vi "infofile beta.vi"(6 "Info in":string[](array[string]), 7 "reference":refnum<vi>) -> (2 "String":string)   [LabVIEW 2020]
uses:
  <vilib>/Utility/Data Type/NI_Data Type.lvlib
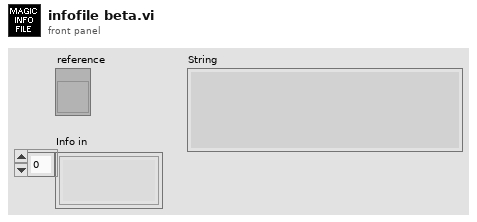
[diagram p1: front panel]
types:
  T1 = typedef "NI_Data Type.lvlib/Data Type.ctl" = enum8{"Invalid Type", "Void", "I8", "I16", "I32", "I64", "U8", "U16", "U32", "U64", "Single Float", "Double Float", "Extended Float", "Single Complex", "Double Complex", "Extended Complex", "Enum U8", "Enum U16", "Enum U32", "Enum U64", "Single Float With Unit", "Double Float With Unit", "Extended Float With Unit", "Single Complex with Unit", "Double Complex with Unit", "Extended Complex with Unit", "Boolean", "String", "Path", "Picture", "Tag", "Array", "Cluster", "Variant", "LV Variant", "Waveform", "Timestamp", "Digital Waveform", "Digital Data", "ExpressData", "Refnum", "External Data", "VI", "Poly VI", "LabVIEW Class Instance", "Fixed Point", "Set Collection", "Map Collection"}
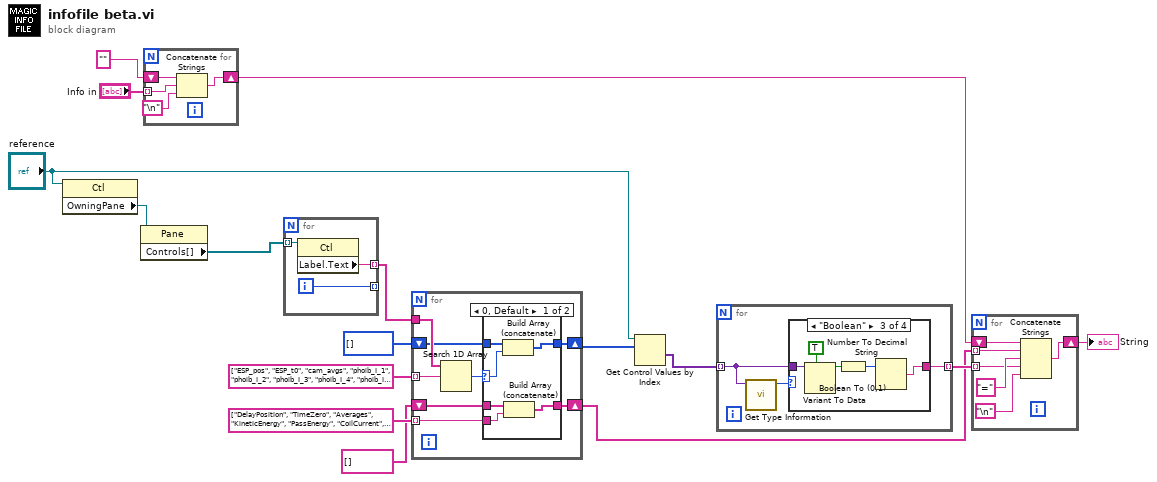
[diagram p0: block diagram]
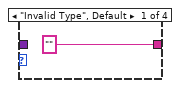
[diagram p2: hidden frame]
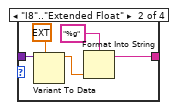
[diagram p3: hidden frame]
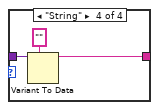
[diagram p4: hidden frame]
diagram:
  n1 = property class="Ctl"(reference="reference") -> ("OwningPane"=w2:refnum<vi>)  [unwired: 1 in, 2 out]
  n2 = property class="Pane"(reference=w2) -> ("Controls[]"=w1:refnum<vi>[])  [unwired: 1 in, 2 out]
  n3 = for {
    tunnel: "Info in" -> [w20] mode=indexing
    shift-right: [w19] -> w11
    shift-left: "" -> [w18]
    n4 = Concatenate Strings(w18, w20, "\n") -> (w19:string)
  }
  n5 = for {
    tunnel: w1 -> [w23] mode=indexing
    tunnel: [w22] -> w13 mode=indexing
    tunnel: [w21] -> _ mode=indexing
    i -> [w21]
    n6 = property class="Ctl"(reference=w23) -> ("Label.Text"=w22:string)  [unwired: 1 in, 2 out]
  }
  n7 = for {
    tunnel: w13 -> [w31]
    tunnel: string[] ["ESP_pos", "ESP_t0", "cam_avgs", "phoib_I_1", "phoib_I_2", "phoib_I_3", "phoib_I_4", "phoib_I_5", "phoib_I_6", "phoib_I_7", "phoib_I_8", "phoib_I_9", "cam_exp", "gain", "binning", "ROI Bottom", "ROI Top", "ROI Right", "ROI Left", "cam_dark?"] -> [w30] mode=indexing
    shift-right: [w28] -> w5
    shift-left: i32[] [] -> [w27]
    tunnel: string[] ["DelayPosition", "TimeZero", "Averages", "KineticEnergy", "PassEnergy", "CoilCurrent", "WorkFunction", "DetectorVoltage", "ScreenVoltage", "ConversionVoltage", "FocusDisplacement1", "FocusDisplacement2", "Exposure", "Gain", "Binning", "ROIbottom", "ROItop", "ROIright", "ROIleft", "DarkImg"] -> [w26] mode=indexing
    shift-right: [w25] -> w8
    shift-left: string[] [] -> [w24]
    n8 = Search 1D Array(1D array=w31, element=w30) -> (index of element=w29:i32)  [unwired: 1 in]
    n9 = case shown="0, Default" w29 {
      selector: w29 -> [w37 _]
      tunnel: [w36 w39] -> w28
      tunnel: w27 -> [w35 w39]
      tunnel: w26 -> [w33 _]
      tunnel: [w32 w38] -> w25
      tunnel: w24 -> [w34 w38]
      frame 0, Default {
        n10 = Build Array (concatenate)(w35, w37) -> (w36:i32[])
        n11 = Build Array (concatenate)(w34, w33) -> (w32:string[])
      }
      frame -1 {
      }
    }
  }
  n12 = Get Control Values by Index(0:"reference", 1:w5) -> (10:w4:variant[])  [unwired: 1 in, 1 out]
  n13 = for {
    tunnel: [w41] -> w15 mode=indexing
    tunnel: w4 -> [w40] mode=indexing
    n14 = call <vilib>:"Get Type Information.vi"("variant"=w40) -> ("type"=w42:T1)  [unwired: 6 in, 4 out]
    n15 = case shown="\"Boolean\"" w42 {
      tunnel: w40 -> [_ w47 w53 w55]
      tunnel: ["" w44 w49 w54] -> w41
      frame "Invalid Type", Default {
      }
      frame "I8".."Extended Float" {
        n16 = Variant To Data(type=ext 0.0, Variant=w47) -> (data=w45:ext)  [unwired: 1 in, 1 out]
        n17 = Format Into String(format string="%g", w45) -> (resulting string=w44:string)  [unwired: 2 in, 1 out]
      }
      frame "Boolean" {
        n18 = Variant To Data(type=TRUE, Variant=w53) -> (data=w51:bool)  [unwired: 1 in, 1 out]
        n19 = Boolean To (0,1)(Boolean=w51) -> (0, 1=w50:i16)
        n20 = Number To Decimal String(number=w50) -> (decimal integer string=w49:string)  [unwired: 1 in]
      }
      frame "String" {
        n21 = Variant To Data(type="", Variant=w55) -> (data=w54:string)  [unwired: 1 in, 1 out]
      }
    }
  }
  n22 = for {
    tunnel: w15 -> [w60] mode=indexing
    tunnel: w8 -> [w62] mode=indexing
    shift-right: [w58] -> w7
    shift-left: w11 -> [w57]
    n23 = Concatenate Strings(w57, w62, "=" ("string"), w60, "\n") -> (w58:string)
  }
  "String" <- w7
